vi "Configure Offset Values.vi"(8 "error in (no error)":errorcluster, 10 "values":dbl[](array[numeric]), 11 "VGC in":refnum<class "PL Inficon VGC.lvclass">) -> (0 "error out":errorcluster, 2 "values":dbl[](array[numeric]), 3 "VGC out":refnum<class "PL Inficon VGC.lvclass">)   [LabVIEW 2015, in "PL Inficon VGC.lvclass"]
doc: "Configures offset values."
uses:
  PL Inficon VGC.lvclass
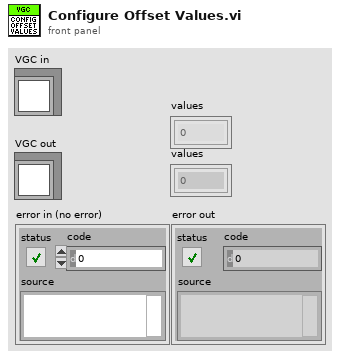
[diagram p1: front panel]
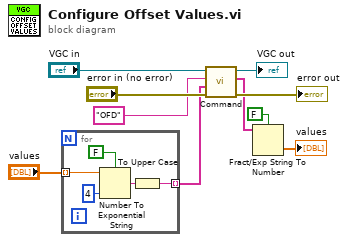
[diagram p0: block diagram]
diagram:
  n1 = for {
    tunnel: "values" -> [w12] mode=indexing
    tunnel: [w11] -> w4 mode=indexing
    n2 = Number To Exponential String(number=w12, precision (6)=i16 4, 1:FALSE ("use system decimal point (T)")) -> (E-format string=w13:string)  [unwired: 1 in]
    n3 = To Upper Case(1:w13) -> (0:w11:string)
  }
  n4 = call "Command.vi"("error in (no error)"="error in (no error)", "parameters"=w4, "command"="OFD" ("format string"), "VGC in"="VGC in") -> ("error out"=→"error out":errorcluster, "response data"=w3:string[], "VGC out"=→"VGC out":refnum<class "PL Inficon VGC.lvclass">)  [unwired: 5 in]
  n5 = Fract/Exp String To Number(use system decimal point (T)=FALSE, string=w3) -> (number=→"values":dbl[])  [unwired: 2 in, 1 out]
